vi "Autonomous.vi"   [LabVIEW 2019]
doc: "This VI starts when autonomous period begins, and will automatically be terminated when it ends. You can carry out timed or sensor driven operations directly to I/O or to subsystems without needing to return to the caller."
uses:
  <vilib>/Rock Robotics/WPI/Utilities/WPI_GetSetVariantRefNum.vi
  <vilib>/Rock Robotics/Network Tables/NT Read String.vi
types:
  T1 = typedef "WPI_JoystickDevRef.ctl" = cluster{"Device":T2}
  T2 = typedef "WPI_JoystickDeviceEnum.ctl" = enum16{"USB 0", "USB 1", "USB 2", "USB 3", "USB 4", "USB 5"}
  T3 = typedef "Command Status Info.ctl" = cluster{"Name":string, "Status":T4, "notifier out":T5}
  T4 = typedef "Completion Status.ctl" = enum16{"Successful", "Aborted", "Incomplete"}
  T5 = typedef "Completion Notifier.ctl" = refnum<notifier>
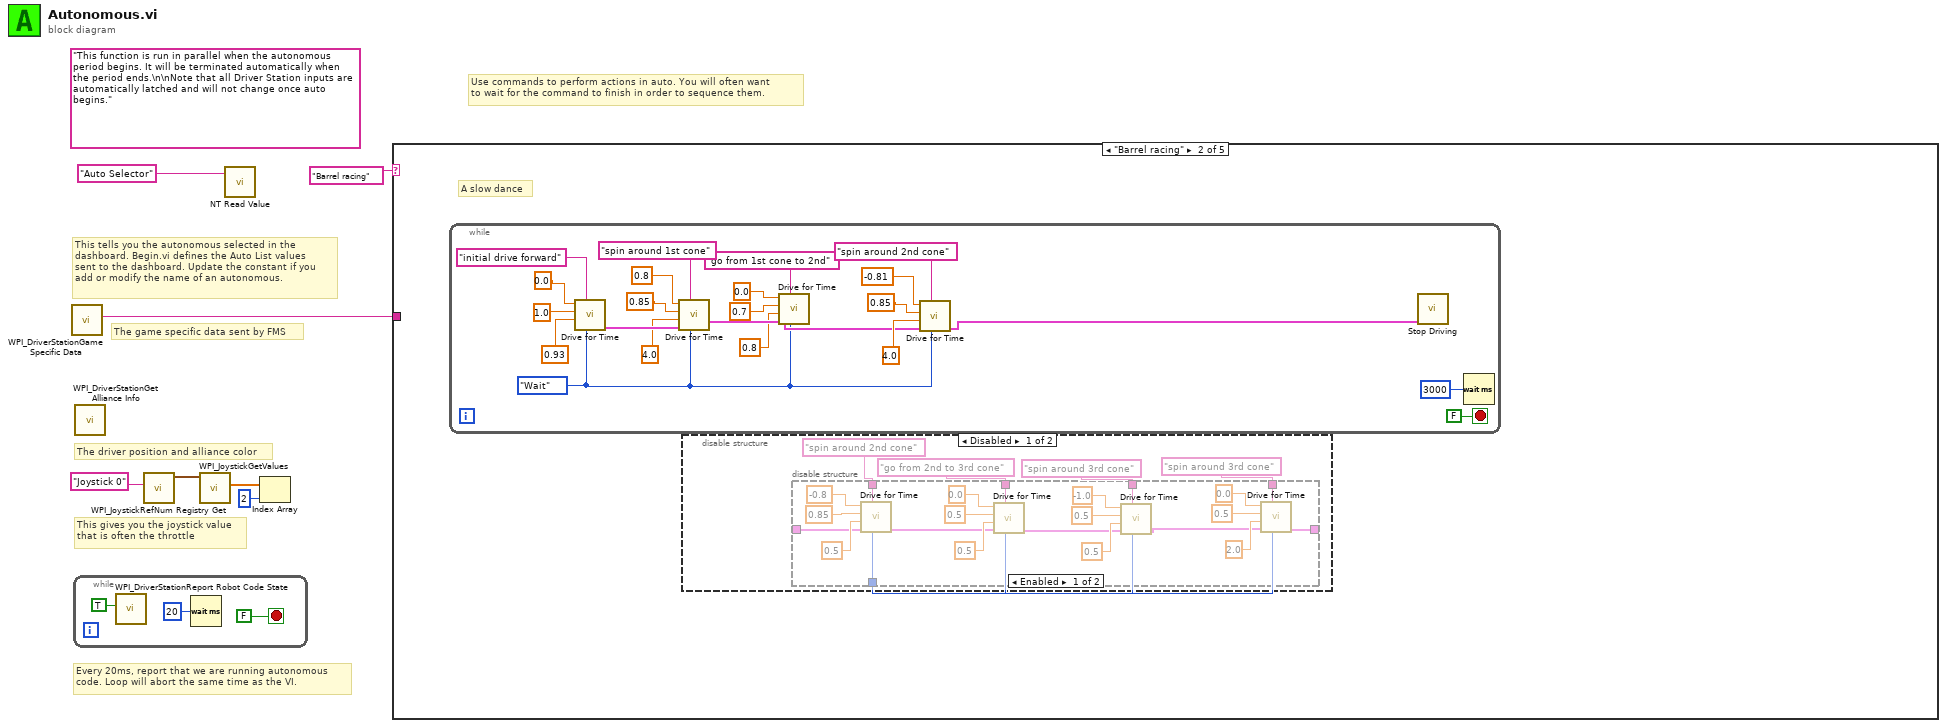
[diagram p0: block diagram]
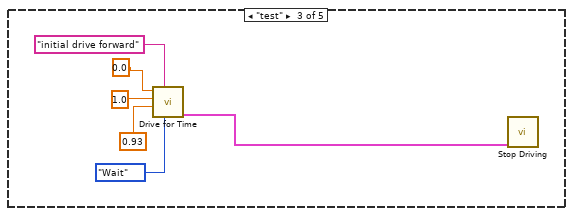
[diagram p5: hidden frame]
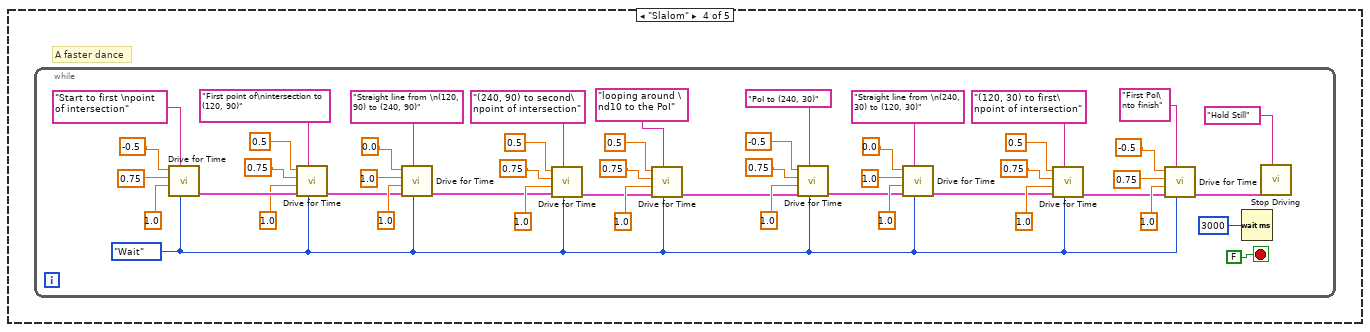
[diagram p6: hidden frame]
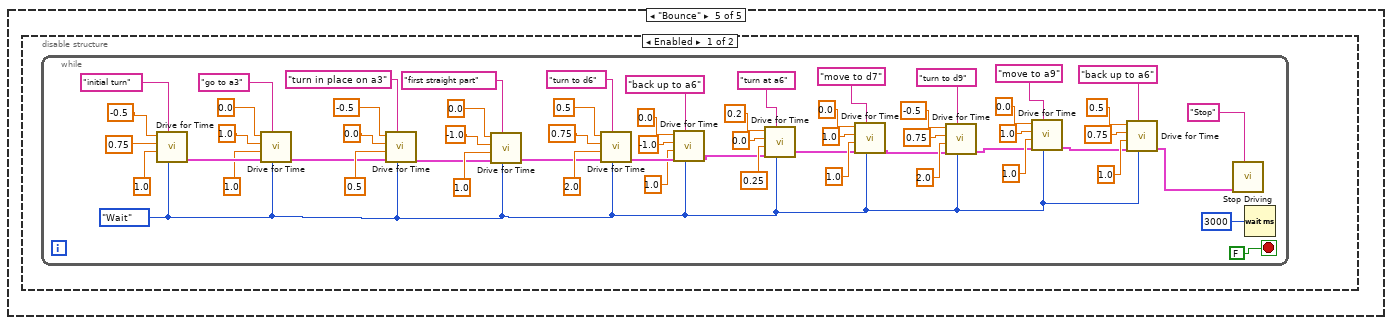
[diagram p7: hidden frame]
diagram:
  (unwired) "This function is run in parallel when the autonomous period begins. It will be terminated automatically when the period ends.\n\nNote that all Driver Station inputs are automatically latched and will not change once auto begins."
  # "The game specific data sent by FMS"
  # "This tells you the autonomous selected in the \ndashboard. Begin.vi defines the Auto List values\nsent to the dashboard. Update the constant if you\nadd or modify the name of an autonomous."
  # "Every 20ms, report that we are running autonomous\ncode. Loop will abort the same time as the VI."
  # "This gives you the joystick value\nthat is often the throttle"
  # "Use commands to perform actions in auto. You will often want\nto wait for the command to finish in order to sequence them."
  # "The driver position and alliance color"
  n1 = call <vilib>:"WPI_DriverStationGame Specific Data.vi"() -> ("Game Specific Data"=w2:string)  [unwired: 11 in]
  n2 = while {
    stop <- FALSE stop-if-true
    n3 = call <vilib>:"WPI_DriverStationReport Robot Code State.vi"("Autonomous"=TRUE) -> ()  [unwired: 10 in, 1 out]
    n4 = Wait (ms)(milliseconds to wait=u32 20) -> ()  [unwired: 1 out]
  }
  n5 = call <vilib>:"WPI_DriverStationGet Alliance Info.vi"() -> ()  [unwired: 12 out]
  n6 = call <vilib>:"WPI_JoystickRefNum Registry Get.vi"("refnum name"="Joystick 0") -> ("JoystickDevRef"=w6:T1)  [unwired: 1 in, 9 out]
  n7 = call <vilib>:"WPI_JoystickGetValues.vi"("JoystickDevRef"=w6) -> ("Axes"=w5:dbl[])  [unwired: 6 in, 4 out]
  n8 = call-poly <vilib>:"NT Read Value.vi"("Name"="Auto Selector") -> ()  [unwired: 9 in, 2 out]
  n9 = Index Array(array=w5, index=2) -> ()  [unwired: 1 out]
  n10 = case shown="\"Barrel racing\"" "Barrel racing" {
    tunnel: w2 -> [_ _ _ _ _]
    frame Default {
      # "You can put your main auto here, or you can right-click on the case and make any\nother frame be the default case."
      # "This is the frame that will execute if no selection is made, or if it is not recognized"
    }
    frame "Barrel racing" {
      # "A slow dance"
      n11 = while {
        stop <- FALSE stop-if-true
        w39 = enum16{"Start", "Wait"}."Wait" ("Synchronication")
        n12 = call "Drive for Time.vi"("Synchronization"=w39, "Description"="initial drive forward", "Seconds"=0.93 ("Delay (s)"), "Joystick y value"=1.0 ("X axis value"), "Joystick x value"=0.0 ("X axis value")) -> ("Command Info Out"=w60:T3)  [unwired: 6 in]
        n13 = call "Drive for Time.vi"("Synchronization"=w39, "Description"="spin around 1st cone", "Command Info In"=w60, "Seconds"=4.0 ("Delay (s)"), "Joystick y value"=0.85 ("X axis value"), "Joystick x value"=0.8 ("X axis value")) -> ("Command Info Out"=w49:T3)  [unwired: 5 in]
        n14 = call "Drive for Time.vi"("Synchronization"=w39, "Description"="go from 1st cone to 2nd", "Command Info In"=w49, "Seconds"=0.8, "Joystick y value"=0.7, "Joystick x value"=0.0) -> ("Command Info Out"=w40:T3)  [unwired: 5 in]
        n15 = call "Drive for Time.vi"("Synchronization"=w39, "Description"="spin around 2nd cone", "Command Info In"=w40, "Seconds"=4.0 ("Delay (s)"), "Joystick y value"=0.85 ("X axis value"), "Joystick x value"=-0.81 ("X axis value")) -> ("Command Info Out"=w38:T3)  [unwired: 5 in]
        n16 = call "Stop Driving.vi"("Command Info In"=w38) -> ()  [unwired: 10 in, 1 out]
        n17 = Wait (ms)(milliseconds to wait=u32 3000 ("millisecond timer value")) -> ()  [unwired: 1 out]
      }
      n18 = disable-structure shown="Disabled" {
        frame Disabled {
          n19 = disable-structure shown="Enabled" {
            disable-tunnel: "spin around 2nd cone" ("Description") -> [w34 _]
            disable-tunnel: _ -> [w33 _]
            disable-tunnel: "go from 2nd to 3rd cone" ("Description") -> [w29 _]
            disable-tunnel: "spin around 3rd cone" ("Description") -> [w24 _]
            disable-tunnel: "spin around 3rd cone" ("Description") -> [w19 _]
            disable-tunnel: [w18 _] -> w11
            disable-tunnel: [w16 _] -> _
            frame Enabled {
              n20 = call "Drive for Time.vi"("Synchronization"=w18, "Description"=w34, "Command Info In"=w33, "Seconds"=0.5, "Joystick y value"=0.85, "Joystick x value"=-0.8) -> ("Command Info Out"=w28:T3)  [unwired: 5 in]
              n21 = call "Drive for Time.vi"("Synchronization"=w18, "Description"=w29, "Command Info In"=w28, "Seconds"=0.5, "Joystick y value"=0.5, "Joystick x value"=0.0) -> ("Command Info Out"=w23:T3)  [unwired: 5 in]
              n22 = call "Drive for Time.vi"("Synchronization"=w18, "Description"=w24, "Command Info In"=w23, "Seconds"=0.5, "Joystick y value"=0.5, "Joystick x value"=-1.0) -> ("Command Info Out"=w17:T3)  [unwired: 5 in]
              n23 = call "Drive for Time.vi"("Synchronization"=w18, "Description"=w19, "Command Info In"=w17, "Seconds"=2.0, "Joystick y value"=0.5, "Joystick x value"=0.0) -> ("Command Info Out"=w16:T3)  [unwired: 5 in]
            }
            frame Disabled {
            }
          }
        }
        frame Enabled {
        }
      }
    }
    frame "test" {
      n24 = call "Drive for Time.vi"("Synchronization"=enum16{"Start", "Wait"}."Wait" ("Synchronication"), "Description"="initial drive forward", "Seconds"=0.93 ("Delay (s)"), "Joystick y value"=1.0 ("X axis value"), "Joystick x value"=0.0 ("X axis value")) -> ("Command Info Out"=w61:T3)  [unwired: 6 in]
      n25 = call "Stop Driving.vi"("Command Info In"=w61) -> ()  [unwired: 10 in, 1 out]
    }
    frame "Slalom" {
      # "A faster dance"
      n26 = while {
        stop <- FALSE stop-if-true
        w69 = enum16{"Start", "Wait"}."Wait" ("Synchronication")
        n27 = call "Drive for Time.vi"("Synchronization"=w69, "Description"="Start to first \npoint of intersection", "Seconds"=1.0 ("Delay (s)"), "Joystick y value"=0.75 ("X axis value"), "Joystick x value"=-0.5 ("X axis value")) -> ("Command Info Out"=w115:T3)  [unwired: 6 in]
        n28 = call "Drive for Time.vi"("Synchronization"=w69, "Description"="First point of\nintersection to (120, 90)", "Command Info In"=w115, "Seconds"=1.0 ("Delay (s)"), "Joystick y value"=0.75 ("X axis value"), "Joystick x value"=0.5 ("X axis value")) -> ("Command Info Out"=w99:T3)  [unwired: 5 in]
        n29 = call "Drive for Time.vi"("Synchronization"=w69, "Description"="Straight line from \n(120, 90) to (240, 90)", "Command Info In"=w99, "Seconds"=1.0 ("Delay (s)"), "Joystick y value"=1.0 ("X axis value"), "Joystick x value"=0.0 ("X axis value")) -> ("Command Info Out"=w95:T3)  [unwired: 5 in]
        n30 = call "Drive for Time.vi"("Synchronization"=w69, "Description"="(240, 90) to second\npoint of intersection", "Command Info In"=w95, "Seconds"=1.0 ("Delay (s)"), "Joystick y value"=0.75 ("X axis value"), "Joystick x value"=0.5 ("X axis value")) -> ("Command Info Out"=w89:T3)  [unwired: 5 in]
        n31 = call "Drive for Time.vi"("Synchronization"=w69, "Description"="looping around \nd10 to the PoI", "Command Info In"=w89, "Seconds"=1.0 ("Delay (s)"), "Joystick y value"=0.75 ("X axis value"), "Joystick x value"=0.5 ("X axis value")) -> ("Command Info Out"=w74:T3)  [unwired: 5 in]
        n32 = call "Drive for Time.vi"("Synchronization"=w69, "Description"="PoI to (240, 30)", "Command Info In"=w74, "Seconds"=1.0 ("Delay (s)"), "Joystick y value"=0.75 ("X axis value"), "Joystick x value"=-0.5 ("X axis value")) -> ("Command Info Out"=w80:T3)  [unwired: 5 in]
        n33 = call "Drive for Time.vi"("Synchronization"=w69, "Description"="Straight line from \n(240, 30) to (120, 30)", "Command Info In"=w80, "Seconds"=1.0 ("Delay (s)"), "Joystick y value"=1.0 ("X axis value"), "Joystick x value"=0.0 ("X axis value")) -> ("Command Info Out"=w76:T3)  [unwired: 5 in]
        n34 = call "Drive for Time.vi"("Synchronization"=w69, "Description"="(120, 30) to first\npoint of intersection", "Command Info In"=w76, "Seconds"=1.0 ("Delay (s)"), "Joystick y value"=0.75 ("X axis value"), "Joystick x value"=0.5 ("X axis value")) -> ("Command Info Out"=w67:T3)  [unwired: 5 in]
        n35 = call "Drive for Time.vi"("Synchronization"=w69, "Description"="First PoI\nto finish", "Command Info In"=w67, "Seconds"=1.0 ("Delay (s)"), "Joystick y value"=0.75 ("X axis value"), "Joystick x value"=-0.5 ("X axis value")) -> ("Command Info Out"=w68:T3)  [unwired: 5 in]
        n36 = Wait (ms)(milliseconds to wait=u32 3000 ("millisecond timer value")) -> ()  [unwired: 1 out]
        n37 = call "Stop Driving.vi"("Description"="Hold Still", "Command Info In"=w68) -> ()  [unwired: 9 in, 1 out]
      }
    }
    frame "Bounce" {
      n38 = disable-structure shown="Enabled" {
        frame Enabled {
          n39 = while {
            stop <- FALSE stop-if-true
            w116 = enum16{"Start", "Wait"}."Wait" ("Synchronication")
            n40 = call "Drive for Time.vi"("Synchronization"=w116, "Description"="initial turn", "Seconds"=1.0 ("Delay (s)"), "Joystick y value"=0.75 ("X axis value"), "Joystick x value"=-0.5 ("X axis value")) -> ("Command Info Out"=w174:T3)  [unwired: 6 in]
            n41 = call "Drive for Time.vi"("Synchronization"=w116, "Description"="go to a3", "Command Info In"=w174, "Seconds"=1.0 ("Delay (s)"), "Joystick y value"=1.0 ("X axis value"), "Joystick x value"=0.0 ("X axis value")) -> ("Command Info Out"=w158:T3)  [unwired: 5 in]
            n42 = call "Drive for Time.vi"("Synchronization"=w116, "Description"="turn in place on a3", "Command Info In"=w158, "Seconds"=0.5 ("Delay (s)"), "Joystick y value"=0.0 ("X axis value"), "Joystick x value"=-0.5 ("X axis value")) -> ("Command Info Out"=w153:T3)  [unwired: 5 in]
            n43 = call "Drive for Time.vi"("Synchronization"=w116, "Description"="first straight part", "Command Info In"=w153, "Seconds"=1.0 ("Delay (s)"), "Joystick y value"=-1.0 ("X axis value"), "Joystick x value"=0.0 ("X axis value")) -> ("Command Info Out"=w148:T3)  [unwired: 5 in]
            n44 = call "Drive for Time.vi"("Synchronization"=w116, "Description"="turn to d6", "Command Info In"=w148, "Seconds"=2.0 ("Delay (s)"), "Joystick y value"=0.75 ("X axis value"), "Joystick x value"=0.5 ("X axis value")) -> ("Command Info Out"=w147:T3)  [unwired: 5 in]
            n45 = call "Drive for Time.vi"("Synchronization"=w116, "Description"="back up to a6", "Command Info In"=w147, "Seconds"=1.0, "Joystick y value"=-1.0, "Joystick x value"=0.0) -> ("Command Info Out"=w138:T3)  [unwired: 5 in]
            n46 = call "Drive for Time.vi"("Synchronization"=w116, "Description"="turn at a6", "Command Info In"=w138, "Seconds"=0.25, "Joystick y value"=0.0, "Joystick x value"=0.2) -> ("Command Info Out"=w133:T3)  [unwired: 5 in]
            n47 = call "Drive for Time.vi"("Synchronization"=w116, "Description"="move to d7", "Command Info In"=w133, "Seconds"=1.0, "Joystick y value"=1.0, "Joystick x value"=0.0) -> ("Command Info Out"=w128:T3)  [unwired: 5 in]
            n48 = call "Drive for Time.vi"("Synchronization"=w116, "Description"="turn to d9", "Command Info In"=w128, "Seconds"=2.0, "Joystick y value"=0.75, "Joystick x value"=-0.5) -> ("Command Info Out"=w123:T3)  [unwired: 5 in]
            n49 = call "Drive for Time.vi"("Synchronization"=w116, "Description"="move to a9", "Command Info In"=w123, "Seconds"=1.0, "Joystick y value"=1.0, "Joystick x value"=0.0) -> ("Command Info Out"=w118:T3)  [unwired: 5 in]
            n50 = call "Drive for Time.vi"("Synchronization"=w116, "Description"="back up to a6", "Command Info In"=w118, "Seconds"=1.0, "Joystick y value"=0.75, "Joystick x value"=0.5) -> ("Command Info Out"=w117:T3)  [unwired: 5 in]
            n51 = call "Stop Driving.vi"("Description"="Stop", "Command Info In"=w117) -> ()  [unwired: 9 in, 1 out]
            n52 = Wait (ms)(milliseconds to wait=u32 3000 ("millisecond timer value")) -> ()  [unwired: 1 out]
          }
        }
        frame Disabled {
        }
      }
    }
  }
